vi "header write.vi"(11 "Which header name":T1) -> (4 "name output":string)   [LabVIEW 2016]
doc: "Writes header file for wheel\ncycle data"
uses:
  realtime data/pixie vis/controls/header name control.ctl
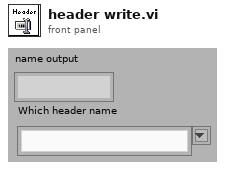
[diagram p1: front panel]
types:
  T1 = typedef "header name control.ctl" = string
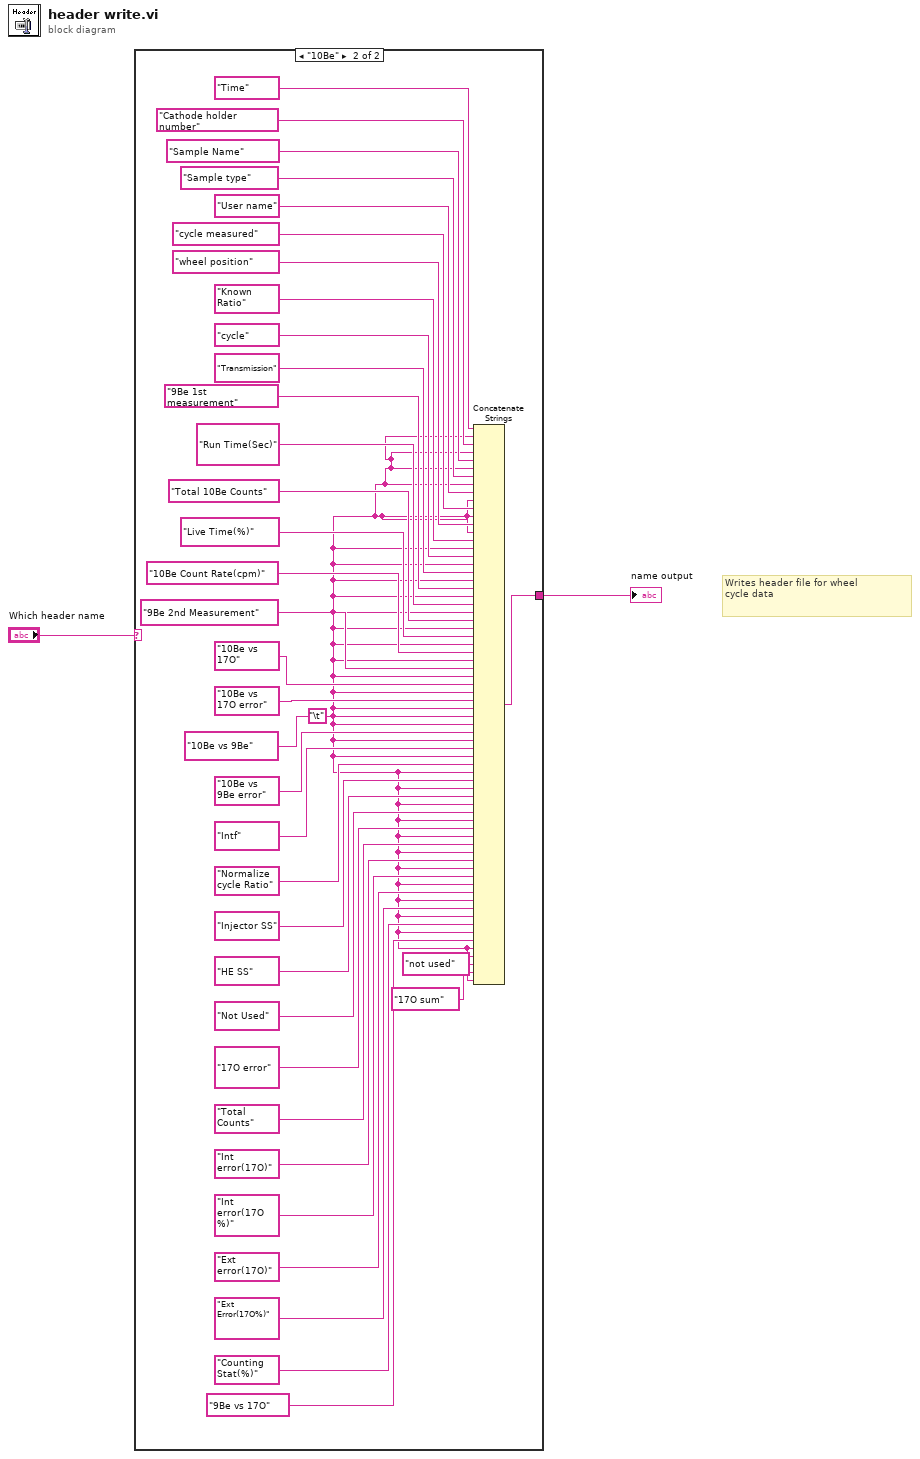
[diagram p0: block diagram]
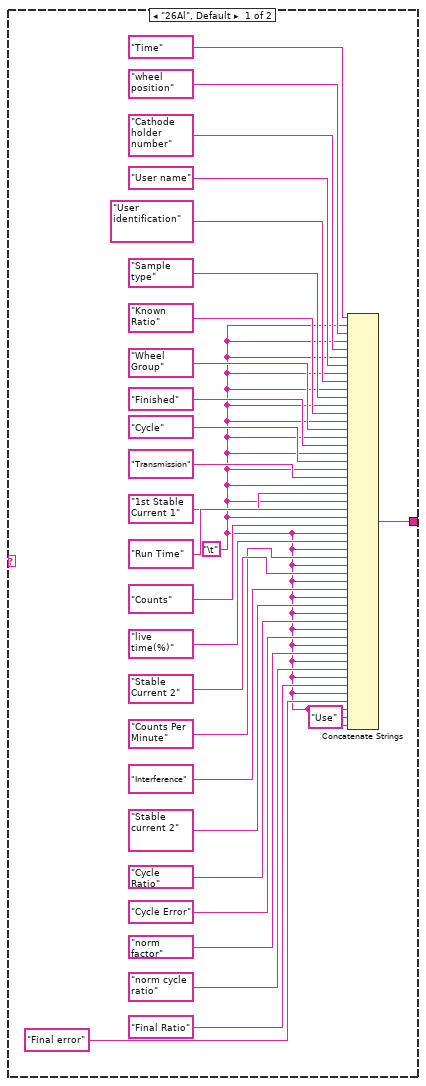
[diagram p2: hidden frame]
diagram:
  # "Writes header file for wheel\ncycle data"
  n1 = case shown="\"10Be\"" "Which header name" {
    tunnel: [w30 w67] -> w2
    frame "26Al", Default {
      w4 = "\t"
      n2 = Concatenate Strings("Time" ("text"), w4, "wheel position" ("text"), w4, "Cathode holder number" ("text"), w4, "User name" ("text"), w4, "User identification" ("text"), w4, "Sample type" ("text"), w4, "Known Ratio" ("text"), w4, "Wheel Group" ("text"), w4, "Finished" ("text"), w4, "Cycle" ("text"), w4, "Transmission" ("text"), w4, "1st Stable Current 1" ("text"), w4, "Run Time" ("text"), w4, "Counts" ("text"), w4, "live time(%)" ("text"), w4, "Counts Per Minute" ("text"), w4, "Stable Current 2" ("text"), w4, "Interference" ("text"), w4, "Stable current 2" ("text"), w4, "Cycle Ratio" ("text"), w4, "Cycle Error" ("text"), w4, "norm factor" ("text"), w4, "norm cycle ratio" ("text"), w4, "Final Ratio" ("text"), w4, "Final error" ("text"), w4, "Use" ("string"), w4) -> (w30:string)
    }
    frame "10Be" {
      w31 = "\t"
      n3 = Concatenate Strings("Time" ("text"), w31, "Cathode holder number" ("text"), w31, "Sample Name" ("text"), w31, "Sample type" ("text"), w31, "User name" ("text"), w31, "cycle measured" ("text"), w31, "wheel position" ("text"), w31, "Known Ratio" ("text"), w31, "cycle" ("text"), w31, "Transmission" ("text"), w31, "9Be 1st measurement" ("text"), w31, "Run Time(Sec)" ("text"), w31, "Total 10Be Counts" ("text"), w31, "Live Time(%)" ("text"), w31, "10Be Count Rate(cpm)" ("text"), w31, "9Be 2nd Measurement" ("text"), w31, "10Be vs 17O" ("text"), w31, "10Be vs 17O error" ("text"), w31, "10Be vs 9Be" ("text"), w31, "10Be vs 9Be error" ("text"), w31, "Intf" ("text"), w31, "Normalize cycle Ratio" ("text"), w31, "Injector SS" ("text"), w31, "HE SS" ("text"), w31, "Not Used" ("text"), w31, "17O error" ("text"), w31, "Total Counts" ("text"), w31, "Int error(17O)" ("text"), w31, "Int error(17O %)" ("text"), w31, "Ext error(17O)" ("text"), w31, "Ext Error(17O%)" ("text"), w31, "Counting Stat(%)" ("text"), w31, "9Be vs 17O" ("string"), w31, "not used" ("string"), w31, "17O sum" ("string"), w31) -> (w67:string)
    }
  }
  "name output" <- w2
